vi "CH_LM App Check Filename.vi"(2 "error in (no error)":errorcluster, 3 "Path":path) -> (0 "error out":errorcluster, 1 "Path":path)   [LabVIEW 2012, in "CH_LM App.lvlib"]
doc: "This VI is used to check for existing files and to renames them by adding/incrementing a number.\n\nExpected filename format: *[_n].*"
uses:
  CH_LM App.lvlib
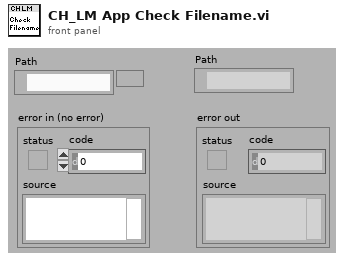
[diagram p1: front panel]
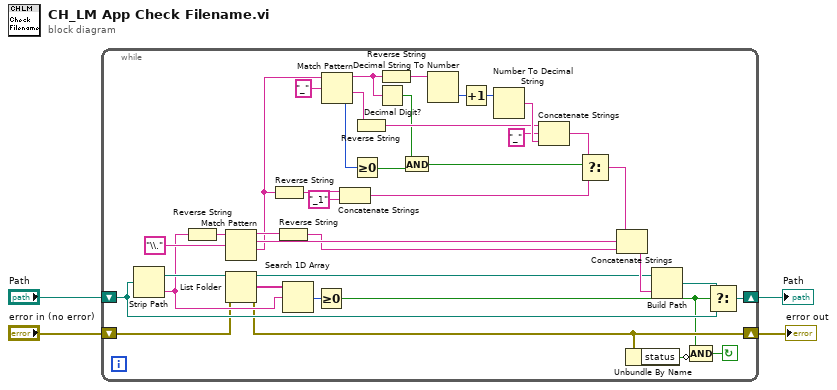
[diagram p0: block diagram]
diagram:
  n1 = while {
    shift-right: [w26] -> w4
    shift-left: "Path" -> [w25]
    shift-right: [w8] -> w1
    shift-left: "error in (no error)" -> [w9]
    stop <- w6 continue-if-true
    n2 = Strip Path(path=w25) -> (stripped path=w12:path, name=w10:string)
    n3 = Reverse String(1:w10) -> (0:w17:string)
    n4 = Match Pattern(string=w17, regular expression="\\.") -> (before substring=w16:string, match substring=w29:string, after substring=w13:string)  [unwired: 2 out]
    n5 = List Folder(path=w12, error in=w9) -> (path out=w11:path, filenames=w23:string[], error out=w8:errorcluster)  [unwired: 3 out]
    n6 = Reverse String(1:w13) -> (0:w14:string)
    n7 = Reverse String(1:w16) -> (0:w15:string)
    n8 = Search 1D Array(1D array=w23, element=w10) -> (index of element=w24:i32)  [unwired: 1 out]
    n9 = Greater Or Equal To 0?(x=w24) -> (x >= 0?=w7:bool)
    n10 = Match Pattern(string=w13, regular expression="_") -> (before substring=w21:string, after substring=w37:string, offset past match=w32:i32)  [unwired: 2 out]
    n11 = Concatenate Strings(w14, "_1" ("string")) -> (w34:string)
    n12 = Greater Or Equal To 0?(x=w32) -> (x >= 0?=w19:bool)
    n13 = Reverse String(1:w37) -> (0:w22:string)
    n14 = Decimal Digit?(1:w21) -> (0:w20:bool)
    n15 = Reverse String(1:w21) -> (0:w35:string)
    n16 = And(x=w20, y=w19) -> (x .and. y?=w18:bool)
    n17 = Decimal String To Number(string=w35) -> (number=w36:i32)  [unwired: 3 out]
    n18 = Increment(x=w36) -> (x+1=w40:i32)
    n19 = Number To Decimal String(number=w40) -> (decimal integer string=w41:string)  [unwired: 1 out]
    n20 = Concatenate Strings(w22, "_" ("string"), w41) -> (w38:string)
    n21 = Select(t=w38, s=w18, f=w34) -> (s? t:f=w42:string)
    n22 = Concatenate Strings(w42, w29, w15) -> (w28:string)
    n23 = Unbundle By Name(w8) -> ("status"=w5:bool)
    n24 = Build Path(base path=w11, name or relative path=w28) -> (appended path=w30:path)
    n25 = Compound Arithmetic op=AND(w7, invert w5) -> (w6:bool)
    n26 = Select(t=w30, s=w7, f=w25) -> (s? t:f=w26:path)
  }
  "Path" <- w4
  "error out" <- w1
